vi "Set PID.vi"(8 "error in (no error)":errorcluster, 10 "PID":T1, 11 "ThermPID in":refnum<class "ThermPID.lvclass">) -> (0 "error out":errorcluster, 3 "ThermPID out":refnum<class "ThermPID.lvclass">)   [LabVIEW 2023, in "ThermPID.lvclass"]
uses:
  ThermPID.lvclass
  PIDController/PIDController.lvclass
  PIDModBus/Controls/Register Enum.ctl
  PIDModBus/PIDModbus.lvlib
  <vilib>/NI/Modbus Library/API/Master/Modbus Master.lvclass
  <userlib>/_OpenG.lib/time/time.llb/openg_time.lvlib
  PIDModBus/Controls/PID Cluster.ctl
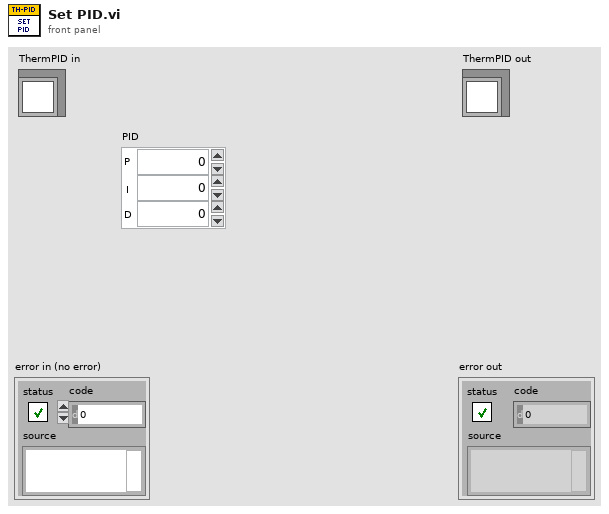
[diagram p1: front panel]
types:
  T1 = typedef "PIDModbus.lvlib/PID Cluster.ctl" = cluster{"P":u16, "I":u16, "D":u16}
  T2 = typedef "PIDModbus.lvlib/Register Enum.ctl" = u16
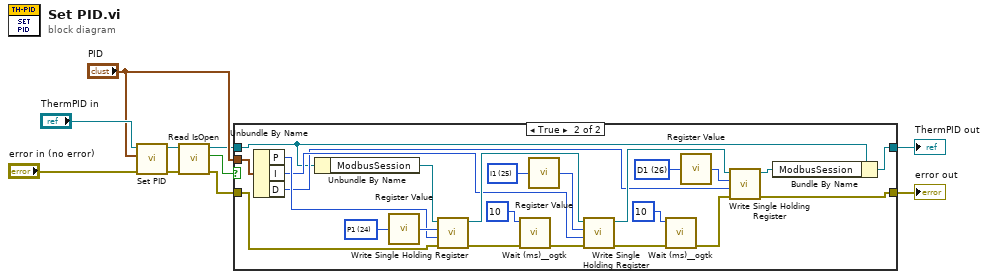
[diagram p0: block diagram]
diagram:
  n1 = call-parent "Set PID.vi"("error in (no error)"="error in (no error)", "PID"="PID", "PIDController in"="ThermPID in") -> ("error out"=w2:errorcluster, "PIDController out"=w7:refnum<class "ThermPID.lvclass">)  [unwired: 7 in]
  n2 = call-dynamic "Read IsOpen.vi"("error in (no error)"=w2, "PIDController in"=w7) -> ("error out"=w3:errorcluster, "IsOpen"=w1:bool, "PIDController out"=w6:refnum<class "ThermPID.lvclass">)  [unwired: 7 in]
  n3 = case shown="True" w1 {
    tunnel: "PID" -> [_ w19]
    tunnel: w6 -> [w12 w17]
    tunnel: [w12 w16] -> w5
    tunnel: [w11 w14] -> w4
    tunnel: w3 -> [w11 w13]
    frame False {
    }
    frame True {
      w28 = T2 26 items=["PV"=0, "SV"=5, "P1"=24, "I1"=25, "D1"=26] ("Register")
      w32 = T2 25 items=["PV"=0, "SV"=5, "P1"=24, "I1"=25, "D1"=26] ("Register")
      w36 = T2 24 items=["PV"=0, "SV"=5, "P1"=24, "I1"=25, "D1"=26] ("Register")
      n4 = Unbundle By Name(w19) -> ("P"=w34:u16, "I"=w26:u16, "D"=w25:u16)
      n5 = Unbundle By Name(w17) -> ("ModbusSession"=w18:refnum<class "Modbus Master.lvclass">)
      n6 = call "Register Value.vi"("Register"=w36) -> ("RegAddr (Hex)"=w35:u16)
      n7 = call-dynamic "Write Single Holding Register.vi"("error in"=w13, "register to write"=w34, "address"=w35, "Modbus master in"=w18) -> ("error out"=w33:errorcluster, "Modbus master out"=w30:refnum<class "Modbus Master.lvclass">)  [unwired: 6 in]
      n8 = call <userlib>:"Wait (ms)__ogtk.vi"("error in (no error)"=w33, "milliseconds to wait"=u32 10) -> ("error out"=w24:errorcluster)  [unwired: 8 in, 1 out]
      n9 = call "Register Value.vi"("Register"=w32) -> ("RegAddr (Hex)"=w31:u16)
      n10 = call-dynamic "Write Single Holding Register.vi"("error in"=w24, "register to write"=w26, "address"=w31, "Modbus master in"=w30) -> ("error out"=w21:errorcluster, "Modbus master out"=w29:refnum<class "Modbus Master.lvclass">)  [unwired: 6 in]
      n11 = call <userlib>:"Wait (ms)__ogtk.vi"("error in (no error)"=w21, "milliseconds to wait"=u32 10) -> ("error out"=w20:errorcluster)  [unwired: 8 in, 1 out]
      n12 = call "Register Value.vi"("Register"=w28) -> ("RegAddr (Hex)"=w27:u16)
      n13 = call-dynamic "Write Single Holding Register.vi"("error in"=w20, "register to write"=w25, "address"=w27, "Modbus master in"=w29) -> ("error out"=w14:errorcluster, "Modbus master out"=w15:refnum<class "Modbus Master.lvclass">)  [unwired: 6 in]
      n14 = Bundle By Name(cluster=w17, "ModbusSession"=w15) -> (w16:refnum<class "ThermPID.lvclass">)
    }
  }
  "error out" <- w4
  "ThermPID out" <- w5
